vi "client.vi"() -> ()   [LabVIEW 2019]
uses:
  Generated_client/RPC Messages/Greeter_req.ctl
  Generated_client/RPC Messages/Greeter_req_req_oneof/Greeter_req_req_oneof.lvclass
  Generated_client/RPC Messages/Greeter_req_req_oneof/Greeter_req_req_oneof.lvclass/Greeter_req_req_oneof.ctl
  Generated_client/RPC Messages/Greeter_res_res_oneof/Greeter_res_res_oneof.lvclass/Greeter_res_res_oneof.ctl
  Generated_client/Generated_client.lvlib
  Generated_client/RPC Messages/Greeter_res_res_oneof/Greeter_res_res_oneof.lvclass
panel:
  out "res_num":i32
  out "res_name":string
  out "res_latitude":i32
  in  "req_latitude":i32
  in  "req_name":string
  in  "req_num":i32
  in  "req_oneof":enum16{"req_name", "req_num"}(ring)
  in  "error in":errorcluster
  out "error out":errorcluster
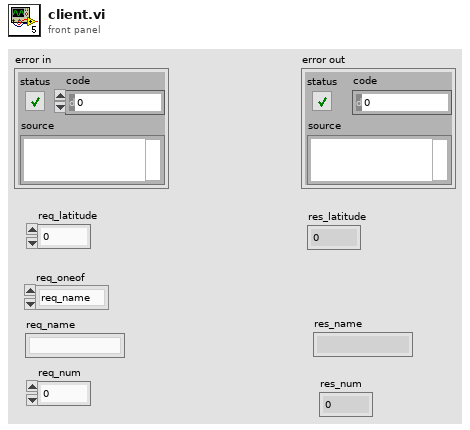
[diagram p1: front panel]
types:
  T1 = typedef "Generated_client.lvlib/Greeter_req.ctl" = cluster{"req_latitude":i32, "Greeter_req_req_oneof":refnum<class "Greeter_req_req_oneof.lvclass">}
  T2 = typedef "grpc-lvsupport-release.lvlib/grpcId.ctl" = u64
  T3 = typedef "Generated_client.lvlib/Greeter_res.ctl" = cluster{"res_latitude":i32, "Greeter_res_res_oneof":refnum<class "Greeter_res_res_oneof.lvclass">}
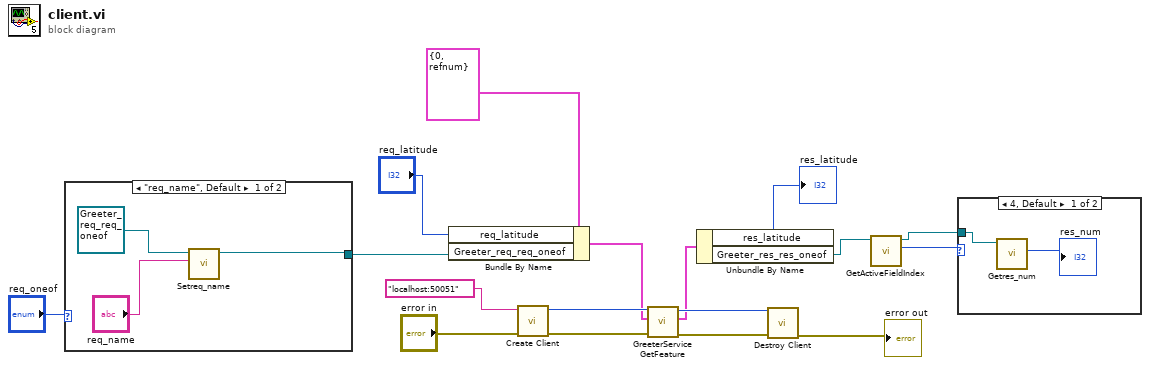
[diagram p0: block diagram]
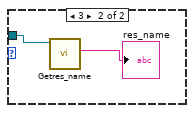
[diagram p2: hidden frame]
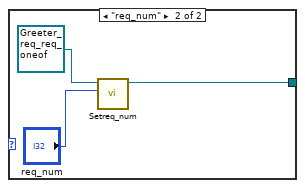
[diagram p3: hidden frame]
diagram:
  n1 = case shown="\"req_name\", Default" "req_oneof" {
    tunnel: [w18 w21] -> w9
    frame "req_name", Default {
      n2 = call "Setreq_name.vi"("Set_Val"="req_name", "OneOfTemplate in"=refnum<class "Greeter_req_req_oneof.lvclass"> refnum) -> ("OneOfTemplate out"=w18:refnum<class "Greeter_req_req_oneof.lvclass">)  [unwired: 8 in, 1 out]
    }
    frame "req_num" {
      n3 = call "Setreq_num.vi"("Set_Val"="req_num", "OneOfTemplate in"=refnum<class "Greeter_req_req_oneof.lvclass"> refnum) -> ("OneOfTemplate out"=w21:refnum<class "Greeter_req_req_oneof.lvclass">)  [unwired: 8 in, 1 out]
    }
  }
  n4 = Bundle By Name(cluster=T1 {"req_latitude"=0, "Greeter_req_req_oneof"=refnum} ("Greeter_req"), "req_latitude"="req_latitude", "Greeter_req_req_oneof"=w9) -> (w8:T1)
  n5 = call "Create Client.vi"("error in"="error in", "address"="localhost:50051") -> ("error out"=w15:errorcluster, "gRPC ID Out"=w17:T2)  [unwired: 8 in]
  n6 = call "GreeterService GetFeature.vi"("error in"=w15, "Request Data"=w8, "gRPC ID"=w17) -> ("error out"=w14:errorcluster, "Response Data"=w7:T3, "gRPC ID out"=w16:T2)  [unwired: 6 in]
  n7 = Unbundle By Name(w7) -> ("res_latitude"=→"res_latitude":i32, "Greeter_res_res_oneof"=w5:refnum<class "Greeter_res_res_oneof.lvclass">)
  n8 = call "Destroy Client.vi"("error in"=w14, "gRPC ID"=w16) -> ("error out"=→"error out":errorcluster)  [unwired: 9 in]
  n9 = call "GetActiveFieldIndex.vi"("OneOfTemplate in"=w5) -> ("Active Field Index"=w4:i32, "OneOfTemplate out"=w3:refnum<class "Greeter_res_res_oneof.lvclass">)  [unwired: 8 in, 1 out]
  n10 = case shown="4, Default" w4 {
    tunnel: w3 -> [w25 w27]
    frame 4, Default {
      n11 = call "Getres_num.vi"("OneOfTemplate in"=w25) -> ("Get_Val"=→"res_num":i32)  [unwired: 8 in, 2 out]
    }
    frame 3 {
      n12 = call "Getres_name.vi"("OneOfTemplate in"=w27) -> ("Get_Val"=→"res_name":string)  [unwired: 8 in, 2 out]
    }
  }
